vi "createColorProjections.vi"(8 "error in (no error)":errorcluster, 9 "spilt ff/fb":bool, 10 "color ims":cluster{"xy im":T1, "xz im":T1, "yz im":T1}, 11 "volumes for display":T3) -> (0 "error out":errorcluster, 3 "color ims out":T2, 4 "ch1 sum":u32, 5 "ch0 sum":u32, 7 "ch0 xy proj sum":u32)   [LabVIEW 2010]
uses:
  <vilib>/vision/Image Controls.llb/IMAQ Image.ctl
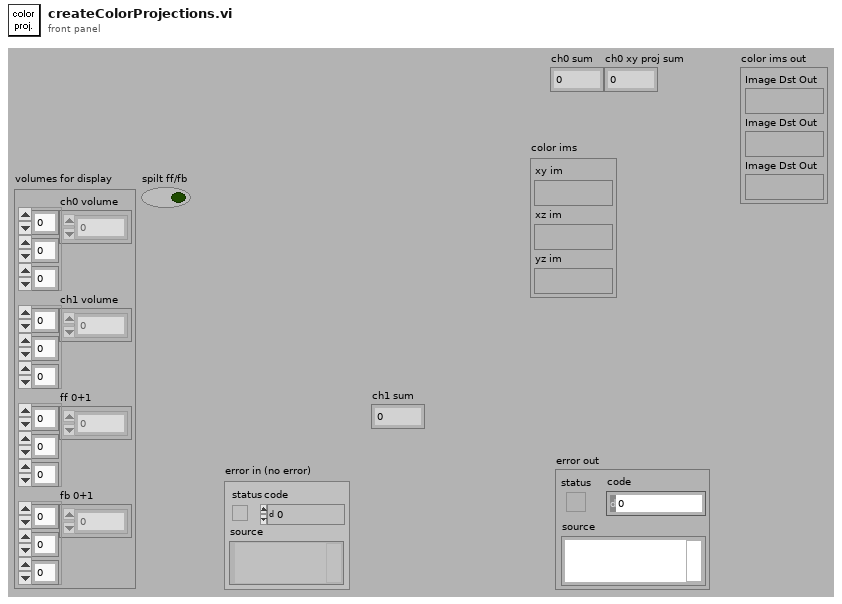
[diagram p1: front panel]
types:
  T1 = typedef "IMAQ Image.ctl" = refnum<image>
  T2 = cluster{"Image Dst Out":T1, "Image Dst Out":T1, "Image Dst Out":T1}
  T3 = cluster{"ch0 volume":u32[][][], "ch1 volume":u32[][][], "ff 0+1":u32[][][], "fb 0+1":u32[][][]}
  T4 = cluster{"Image Out":T1, "Image Out":T1, "Image Out":T1}
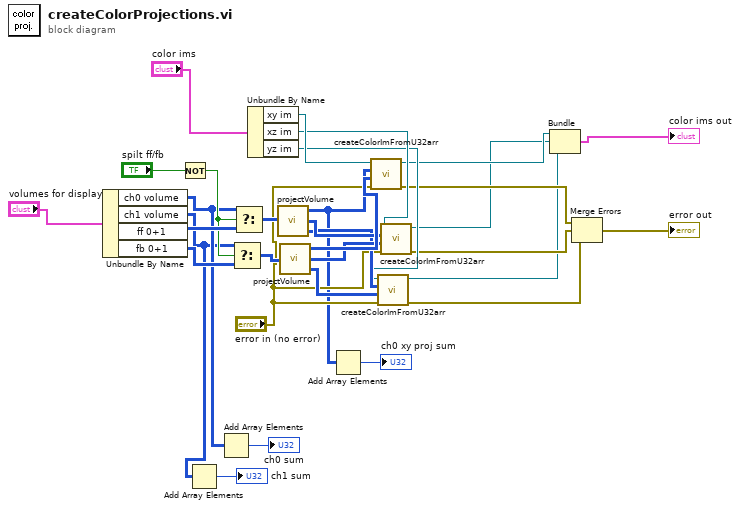
[diagram p0: block diagram]
diagram:
  n1 = Unbundle By Name("volumes for display") -> ("ch0 volume"=w23:u32[][][], "ch1 volume"=w20:u32[][][], "ff 0+1"=w29:u32[][][], "fb 0+1"=w26:u32[][][])
  n2 = Not(x="spilt ff/fb") -> (.not. x?=w27:bool)
  n3 = Add Array Elements(numeric array=w20) -> (sum=→"ch1 sum":u32)
  n4 = Add Array Elements(numeric array=w23) -> (sum=→"ch0 sum":u32)
  n5 = Select(t=w20, s=w27, f=w26) -> (s? t:f=w24:u32[][][])
  n6 = Select(t=w23, s=w27, f=w29) -> (s? t:f=w25:u32[][][])
  n7 = Unbundle By Name("color ims") -> ("xy im"=w13:T1, "xz im"=w12:T1, "yz im"=w11:T1)
  n8 = call "projectVolume.vi"("input array"=w25) -> ("YZ view"=w16:u32[][], "XZ view"=w18:u32[][], "XY view"=w2:u32[][])
  n9 = call "projectVolume.vi"("input array"=w24) -> ("YZ view"=w15:u32[][], "XZ view"=w17:u32[][], "XY view"=w19:u32[][])
  n10 = Add Array Elements(numeric array=w2) -> (sum=→"ch0 xy proj sum":u32)
  n11 = call "createColorImFromU32arr.vi"("error in (no error)"="error in (no error)", "g buffer"=w19, "r buffer"=w2, "Image"=w13) -> ("error out"=w10:errorcluster, "Image Out"=w7:T1)  [unwired: 6 in]
  n12 = call "createColorImFromU32arr.vi"("error in (no error)"="error in (no error)", "g buffer"=w15, "r buffer"=w16, "Image"=w11) -> ("error out"=w8:errorcluster, "Image Out"=w5:T1)  [unwired: 6 in]
  n13 = call "createColorImFromU32arr.vi"("error in (no error)"="error in (no error)", "g buffer"=w17, "r buffer"=w18, "Image"=w12) -> ("error out"=w9:errorcluster, "Image Out"=w6:T1)  [unwired: 6 in]
  n14 = Bundle("Image Out"=w7, "Image Out"=w6, "Image Out"=w5) -> (→"color ims out":T4)  [unwired: 1 in]
  n15 = Merge Errors(w10, w9, w8) -> (→"error out":errorcluster)
